vi "Snap.vi"(8 "error in (no error)":errorcluster, 11 "Vision in":refnum<class "Vision.lvclass">) -> (0 "error out":errorcluster, 3 "Vision out":refnum<class "Vision.lvclass">)   [LabVIEW 2021, in "Vision.lvlib" / "Vision.lvclass"]
uses:
  Vision.lvclass
  C:/Program Files (x86)/National Instruments/LabVIEW 2021/vi.lib/ActorFramework/Actor/Actor.lvclass
  Vision.lvclass/Vision.ctl
  <vilib>/vision/driver/IMAQdx.llb/IMAQdx Buffer Number Mode.ctl
  <vilib>/ActorFramework/Actor/Actor.lvclass/Actor.ctl
  <vilib>/ActorFramework/Message Enqueuer/Message Enqueuer.lvclass/Message Enqueuer.ctl
  7f453908-9464-42ab-bd8f-d2c0393c8175.vi
  <vilib>/ActorFramework/Message Enqueuer/Init from Existing Queue.vi
  <vilib>/ActorFramework/Message Enqueuer/Enqueue.vi
  Vision Messages/Snap Msg/Snap Msg.lvclass
  C:/Program Files (x86)/National Instruments/LabVIEW 2021/vi.lib/ActorFramework/Message/Message.lvclass
  <vilib>/ActorFramework/Message Priority Queue/Priority Enqueue.vi
  <vilib>/ActorFramework/Message Enqueuer/Message Enqueuer.lvclass
  <vilib>/vision/driver/NI_Vision_Acquisition_Software.lvlib
  <vilib>/ActorFramework/Actor/Actor.lvclass
panel:
  out "save":u32
  out "total":u32
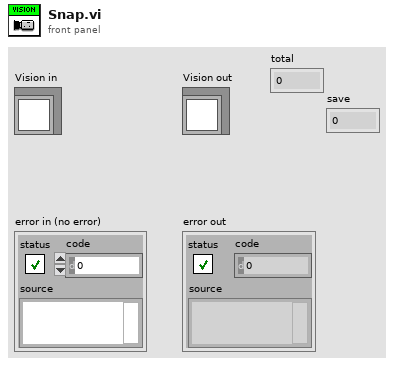
[diagram p1: front panel]
types:
  T1 = typedef "NI_Vision_Acquisition_Software.lvlib/IMAQdx Buffer Number Mode.ctl" = enum32{"Next", "Last", "Buffer Number", "Every", "Last New"}
  T2 = typedef "IMAQdx.ctl" = refnum<k21>
  T3 = typedef "IMAQ Image.ctl" = refnum<image>
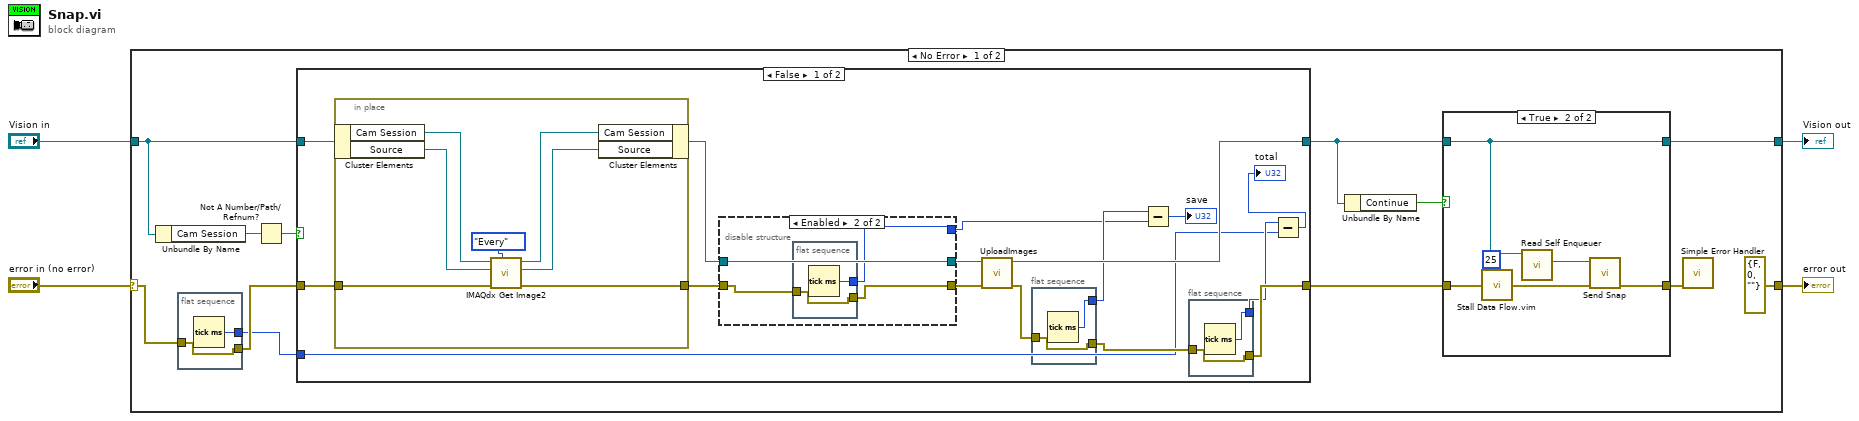
[diagram p0: block diagram]
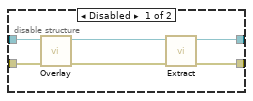
[diagram p2: hidden frame]
diagram:
  n1 = case shown="No Error" "error in (no error)" {
    selector: "error in (no error)" -> [w13 w69]
    tunnel: [errorcluster {"status"=FALSE, "code"=0, "source"=""} ("error IO") w69] -> w3
    tunnel: [w7 w68] -> w1
    tunnel: "Vision in" -> [w5 w68]
    frame No Error {
      n2 = Unbundle By Name(w5) -> ("Cam Session"=w16:T2)
      n3 = flat-sequence {
        tunnel: w13 -> [w18]
        tunnel: [w18] -> w12
        tunnel: [w17] -> w11
        frame #0 {
          n4 = Tick Count (ms)() -> (millisecond timer value=w17:u32)
        }
      }
      n5 = Not A Number/Path/Refnum?(number/path/refnum=w16) -> (NaN/Path/Refnum?=w15:bool)
      n6 = case shown="False" w15 {
        tunnel: w12 -> [w34 w58]
        tunnel: [w31 w59] -> w8
        tunnel: [w30 w58] -> w9
        tunnel: w5 -> [w33 w59]
        tunnel: w11 -> [w26 _]
        frame False {
          n7 = in-place {
            in-place-border: w34 -> [w54]
            in-place-border: [w53] -> w22
            n8 = in-place-cluster #1(w33) -> ("Cam Session"=w57:T2, "Source"=w56:T3)
            n9 = call <vilib>:"IMAQdx Get Image2.vi"("Buffer Number Mode (Next)"=IMAQdx_Buffer_Number_Mode."Every", "error in"=w54, "Image In"=w56, "Session In"=w57) -> ("error out"=w53:errorcluster, "Image Out"=w51:T3, "Session Out"=w52:T2)  [unwired: 4 in, 1 out]
            n10 = in-place-cluster #1("Cam Session"=w52, "Source"=w51) -> (w23:refnum<class "Vision.lvclass">)
          }
          n11 = disable-structure shown="Enabled" {
            disable-tunnel: [w40 w44] -> w32
            disable-tunnel: w23 -> [w39 w44]
            disable-tunnel: w22 -> [w37 w43]
            disable-tunnel: [w35 w42] -> w21
            disable-tunnel: [_ w41] -> w20
            frame Disabled {
              n12 = call "Overlay.vi"("error in (no error)"=w37, "Vision in"=w39) -> ("error out"=w36:errorcluster, "Vision out"=w38:refnum<class "Vision.lvclass">)  [unwired: 8 in]
              n13 = call-dynamic "Extract.vi"("error in (no error)"=w36, "Vision in"=w38) -> ("error out"=w35:errorcluster, "Vision out"=w40:refnum<class "Vision.lvclass">)  [unwired: 8 in]
            }
            frame Enabled {
              n14 = flat-sequence {
                tunnel: w43 -> [w46]
                tunnel: [w46] -> w42
                tunnel: [w45] -> w41
                frame #0 {
                  n15 = Tick Count (ms)() -> (millisecond timer value=w45:u32)
                }
              }
            }
          }
          n16 = call "UploadImages.vi"("error in (no error)"=w21, "Vision in"=w32) -> ("error out"=w19:errorcluster, "Vision out"=w31:refnum<class "Vision.lvclass">)  [unwired: 8 in]
          n17 = flat-sequence {
            tunnel: w19 -> [w48]
            tunnel: [w48] -> w27
            tunnel: [w47] -> w25
            frame #0 {
              n18 = Tick Count (ms)() -> (millisecond timer value=w47:u32)
            }
          }
          n19 = Subtract(x=w25, y=w20) -> (x-y=→"save":u32)
          n20 = flat-sequence {
            tunnel: w27 -> [w50]
            tunnel: [w50] -> w30
            tunnel: [w49] -> w29
            frame #0 {
              n21 = Tick Count (ms)() -> (millisecond timer value=w49:u32)
            }
          }
          n22 = Subtract(x=w29, y=w26) -> (x-y=→"total":u32)
        }
        frame True {
        }
      }
      n23 = Unbundle By Name(w8) -> ("Continue"=w10:bool)
      n24 = case shown="True" w10 {
        tunnel: w9 -> [w60 w65]
        tunnel: w8 -> [w61 w67]
        tunnel: [w61 w67] -> w7
        tunnel: [w60 w64] -> w6
        frame False {
        }
        frame True {
          n25 = call "Stall Data Flow.vim"("value in"=w65, "milliseconds to wait"=u32 25) -> ("value out"=w63:errorcluster)  [unwired: 1 out]
          n26 = call <vilib>:"Read Self Enqueuer.vi"("Actor"=w67) -> ("Self Enqueuer"=w66:refnum<class "Message Enqueuer.lvclass">)  [unwired: 10 in]
          n27 = call "Send Snap.vi"("error in (no error)"=w63, "Message Enqueuer"=w66) -> ("error out"=w64:errorcluster)  [unwired: 8 in, 1 out]
        }
      }
      n28 = call <vilib>:"Simple Error Handler.vi"("error in (no error)"=w6) -> ()  [unwired: 4 in, 5 out]
    }
    frame Error {
    }
  }
  "error out" <- w3
  "Vision out" <- w1
